vi "Read_notifier_data.vi"(0 "DVR Notifier in":refnum<data-value>, 11 "error in (no error)":errorcluster) -> (4 "DVR Notifier out":refnum<data-value>, 6 "DATA":T1, 15 "error out":errorcluster)   [LabVIEW 2020, in "Notifiers.lvclass"]
doc: "Read data to notifier."
uses:
  Classes/Children/Intra-Application/Children/With Data/Children/Notifiers/Notifiers.lvclass
  Classes/Children/Intra-Application/Children/With Data/Children/Notifiers/Notifiers.lvclass/Notifiers.ctl
  Accessors/Read/Read DATA_Notifiers.vi
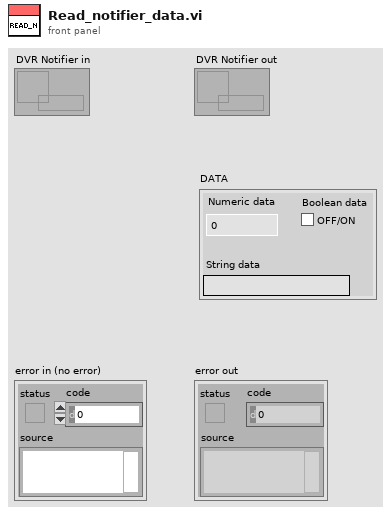
[diagram p1: front panel]
types:
  T1 = cluster{"Numeric data":dbl, "String data":string, "Boolean data":bool}
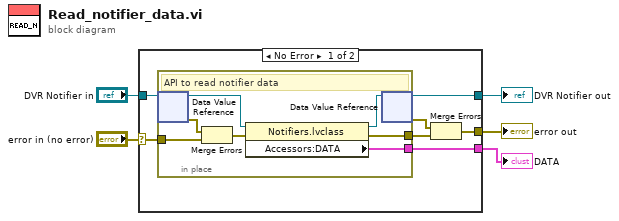
[diagram p0: block diagram]
diagram:
  n1 = case shown="No Error" "error in (no error)" {
    selector: "error in (no error)" -> [w12 w21]
    tunnel: [w9 w21] -> w4
    tunnel: [w8 _] -> w1
    tunnel: "DVR Notifier in" -> [w7 w20]
    tunnel: [w6 w20] -> w2
    frame No Error {
      n2 = in-place "In Place Element Structure" {
        in-place-border: [w17] -> w11
        in-place-border: w12 -> [w15]
        in-place-border: [w13] -> w8
        # "API to read notifier data"
        n3 = in-place-dvr #1(w7) -> (w16:refnum<class "Notifiers.lvclass">, w19:errorcluster)
        n4 = Merge Errors(w19, w15) -> (w18:errorcluster)
        n5 = property on="Property Node" class="Notifiers.lvclass"(reference=w16, error in=w18) -> (reference out=w14:refnum<class "Notifiers.lvclass">, error out=w17:errorcluster, "Accessors:DATA"=w13:T1)
        n6 = in-place-dvr #1(w14) -> (w6:refnum<data-value>, w10:errorcluster)
      }
      n7 = Merge Errors(w10, w11) -> (w9:errorcluster)
    }
    frame Error {
    }
  }
  "error out" <- w4
  "DVR Notifier out" <- w2
  "DATA" <- w1
